vi "Complex IIR Filter (complex signal).vi"(2 "init/cont (init:F)":bool, 3 "Forward Coefficients":cdb[](array[numeric]), 4 "Reverse Coefficients":cdb[](array[numeric]), 5 "X":cdb[](array[numeric])) -> (0 "error":i32, 1 "Filtered X":cdb[](array[numeric]))   [LabVIEW 2020, in "NI_AALBase.lvlib"]
uses:
  NI_AALBase.lvlib
  <resource>/lvanlys.dll
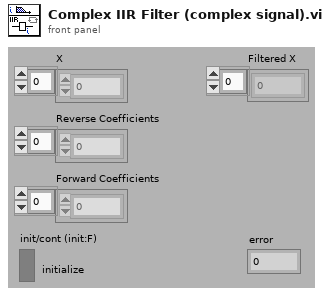
[diagram p1: front panel]
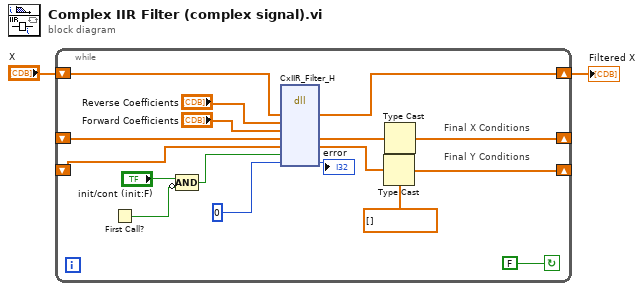
[diagram p0: block diagram]
diagram:
  n1 = while {
    shift-left: _ -> [w11]
    shift-right: [w18] -> _
    shift-left: _ -> [w3]
    shift-right: [w19] -> _
    shift-right: [w6] -> w1
    shift-left: "X" -> [w7]
    stop <- FALSE continue-if-true
    w17 = cdb[] [] ("type for the shift register")
    # "Final Y Conditions"
    # "Final X Conditions"
    n2 = First Call?() -> (First Call?: T/F=w4:bool)
    n3 = Compound Arithmetic op=AND("init/cont (init:F)", invert w4) -> (w5:bool)
    n4 = dll-call lib="C:/Program Files (x86)/National Instruments/LabVIEW 2020/resource/lvanlys.*" fn="CxIIR_Filter_H"("X"=w7, "Reverse Coefficients"="Reverse Coefficients", "Forward Coefficients"="Forward Coefficients", "type for the shift register"=w3, "type for the shift register"=w11, w5, "dsperr"=0) -> ("X"=w6:cdb[], "type for the shift register"=w12:cdb[], "type for the shift register"=w10:cdb[], "dsperr"=→"error":i32)  [unwired: 7 in, 2 out]
    n5 = Type Cast(type=w17, x=w10) -> (*(type *) &x=w18:cdb[])
    n6 = Type Cast(type=w17, x=w12) -> (*(type *) &x=w19:cdb[])
  }
  "Filtered X" <- w1
